vi "ShowIQvaluesAsync.vi"(11 "IQ data":dbl[][](array[numeric])) -> ()   [LabVIEW 2013]
panel:
  in  "error in (no error)":errorcluster
  out "error out":errorcluster
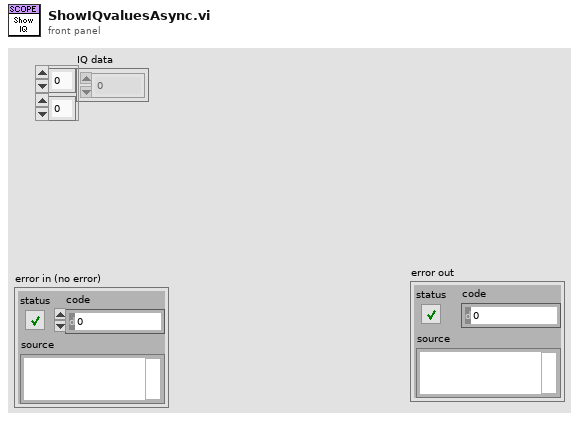
[diagram p1: front panel]
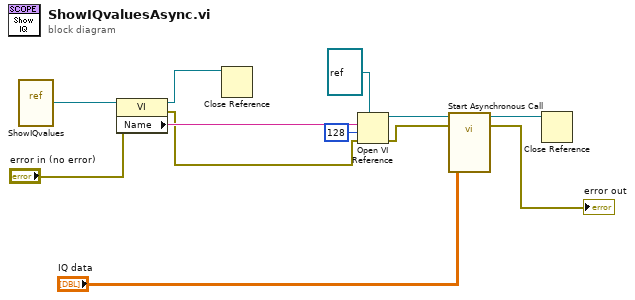
[diagram p0: block diagram]
diagram:
  n1 = vi-ref "ShowIQvalues.vi"() -> (w11:refnum<vi>)
  n2 = property class="VI"(reference=w11, error in="error in (no error)") -> (reference out=w7:refnum<vi>, error out=w5:errorcluster, "Name"=w10:string)
  n3 = Close Reference(reference=w7) -> ()  [unwired: 1 in, 1 out]
  n4 = Open VI Reference(type specifier VI Refnum (for type only)=refnum<vi> refnum, vi path=w10, options=128, error in (no error)=w5) -> (vi reference=w8:refnum<vi>, error out=w4:errorcluster)  [unwired: 2 in]
  n5 = call-by-ref "Start Asynchronous Call"(reference=w8, error in=w4, "Waveform Graph"="IQ data") -> (reference out=w6:refnum<vi>, error out=→"error out":errorcluster)  [unwired: 11 in]
  n6 = Close Reference(reference=w6) -> ()  [unwired: 1 in, 1 out]
